vi "NI VeriStand - Add Custom Device Waveform.vi"(4 "Property Values":variant[](array[variant]), 5 "Highlight? (F)":bool, 6 "Property names":string[](array[string]), 7 "GUID (Default Waveform)":string="83F792DC-AED3-09DF-CB38-512C04DA274D", 8 "error in (no error)":errorcluster, 9 "Waveform":T2, 10 "Waveform Name":string, 11 "Parent Ref in":T1 format="%.0x") -> (0 "error out":errorcluster, 1 "Waveform Ref":T1 format="%.0x", 2 "Newly Created?":bool, 3 "Parent Ref out":T1 format="%.0x")   [LabVIEW 2020, in "Custom Device API.lvlib"]
doc: "Adds a waveform item to the device or device subsection specified by <B>Parent Ref in</B>. If the <B>Waveform Name</B> you specify already exists, this VI updates the <B>Waveform</B> information (<B>Data Type</B>, <B>Units</B>, etc.), properties, and the <B>GUID</B> for the configuration page."
uses:
  <vilib>/NI VeriStand/Custom Device API/Custom Device API.lvlib
  <vilib>/NI VeriStand/Custom Device API/Custom Device Item Ref.ctl
  <vilib>/NI VeriStand/Custom Device API/Custom Device Waveform.ctl
  <vilib>/NI VeriStand/Custom Device API/Custom Device Waveform DataType.ctl
  5c0096cd-a35f-4cc2-9bdd-4f083383587a.vi
  <vilib>/NI VeriStand/Custom Device API/Custom Device Offline Path.vi
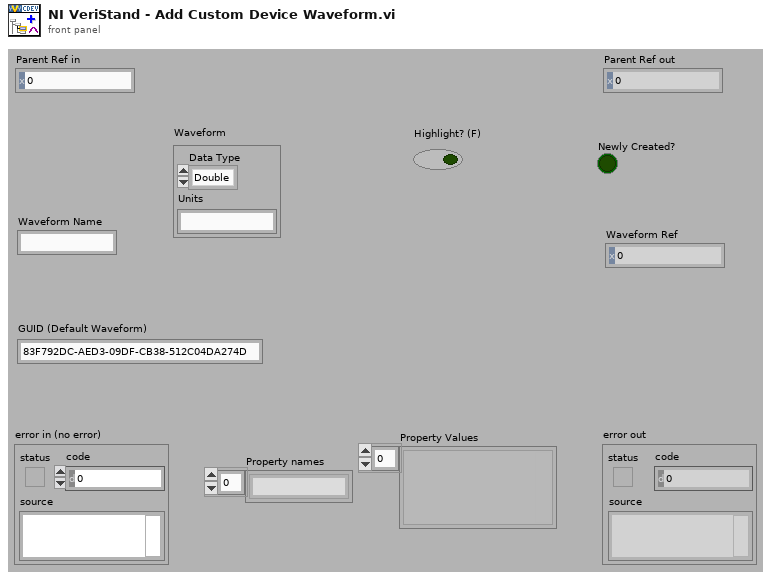
[diagram p1: front panel]
types:
  T1 = typedef "Custom Device API.lvlib/Custom Device Item Ref.ctl" = u64
  T2 = typedef "Custom Device API.lvlib/Custom Device Waveform.ctl" = cluster{"Data Type":T3, "Units":string}
  T3 = typedef "Custom Device API.lvlib/Custom Device Waveform DataType.ctl" = enum16{"Double", "Complex Double"}
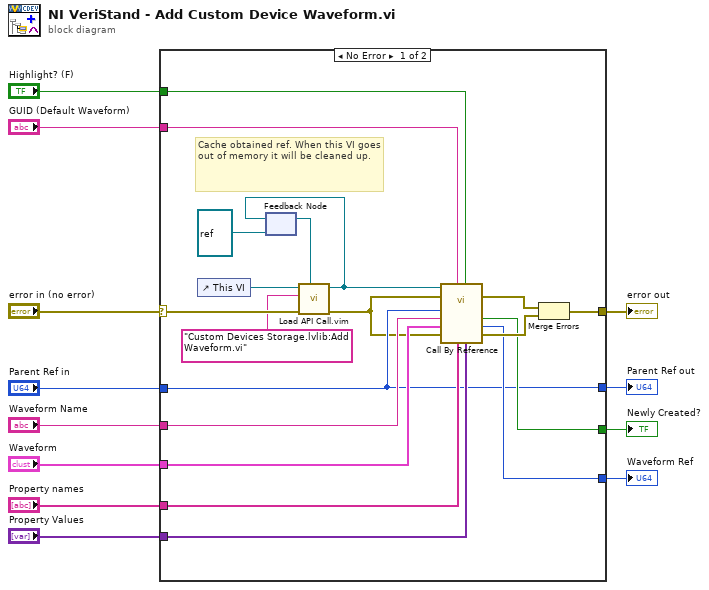
[diagram p0: block diagram]
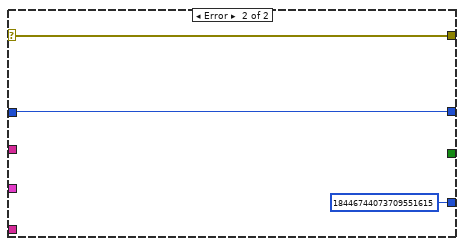
[diagram p2: hidden frame]
diagram:
  n1 = case shown="No Error" "error in (no error)" {
    selector: "error in (no error)" -> [w17 w34]
    tunnel: "GUID (Default Waveform)" -> [w30 _]
    tunnel: "Highlight? (F)" -> [w29 _]
    tunnel: [w28 T1 18446744073709551615 ("Channel Ref")] -> w10
    tunnel: [w27 w34] -> w9
    tunnel: [w20 w32] -> w8
    tunnel: "Property Values" -> [w26 _]
    tunnel: "Property names" -> [w25 _]
    tunnel: "Parent Ref in" -> [w20 w32]
    tunnel: "Waveform Name" -> [w24 _]
    tunnel: "Waveform" -> [w23 _]
    tunnel: [w22 _] -> w2
    frame No Error {
      # "Cache obtained ref. When this VI goes out of memory it will be cleaned up."
      n2 = control-ref of="This VI"() -> (w18:refnum<vi>)
      n3 = feedback #1(refnum<vi> refnum ("type specifier VI Refnum (for type only)")) -> (w19:refnum<vi>)
      n4 = call "Load API Call.vim"("VI reference in"=w19, "error in (no error)"=w17, "VI qualified name"="Custom Devices Storage.lvlib:Add Waveform.vi", "Caller VI ref"=w18) -> ("error out"=w14:errorcluster, "VI reference"=w16:refnum<vi>)  [unwired: 6 in]
      n5 = feedback-in #1(w16) -> ()
      n6 = call-by-ref "?"(reference=w16, error in=w14, "Property Values"=w26, "Highlight? (F)"=w29, "Property names"=w25, "GUID (Default Waveform)"=w30, 8:"error in (no error)"=w14, "Waveform"=w23, "Waveform Name"=w24, "Parent Ref in"=w20) -> (error out=w21:errorcluster, 0:"error out"=w31:errorcluster, "Waveform Ref"=w28:T1, "Newly Created?"=w22:bool)  [unwired: 2 out]
      n7 = Merge Errors(w21, w31) -> (w27:errorcluster)
    }
    frame Error {
    }
  }
  "Parent Ref out" <- w8
  "error out" <- w9
  "Waveform Ref" <- w10
  "Newly Created?" <- w2
